vi "OutputActuators.vi"   [LabVIEW 2020]
uses:
  <vilib>/Rock Robotics/WPI/Solenoid/WPI_SolenoidValue.ctl
  cb7c92a0-f2e0-4add-9935-f208a2f5d3d6.vi
  dfd904db-942a-4b3e-8a93-2d5956c08777.vi
  05c4d3af-9fca-48dd-b3f9-451663aedd7e.vi
  outputs.vi
  TAI_Solenoid.vi
  dsdata.vi
  refnums.vi
  GRNF_GenericSolenoid.vi
  <vilib>/Rock Robotics/WPI/Solenoid/WPI_SolenoidSetEnum.vi
  <vilib>/Rock Robotics/WPI/ThirdParty/Phoenix-LabVIEW/Motor Controller/Controls/CTRE_Phoenix_MotorControl_ControlMode.ctl
  dbda877a-b90e-4fd7-958b-38a76fa4c161.vi
  GRNF_CTREMotor.vi
  TAI_Motor.vi
  cd96a094-93cf-4b37-bace-1743d092b962.vi
  3743a8f9-5793-4711-a231-b942b815bc77.vi
  c5faff8a-f8d6-4d9e-b396-3937cb23a7d4.vi
types:
  T1 = typedef "CTRE_Phoenix_MotorControl_ControlMode.ctl" = u16
  T2 = typedef "WPI_MotorControlDeviceRef.ctl" = cluster{"DeviceStatus":errorcluster, "Type":T3, "PWM":cluster{"PWM Channel":T4, "DeadBand":T5}, "CAN":cluster{"Device Number":u8, "SetOutput VI Ref":variant, "GetOutput VI Ref":variant, "Enable VI Ref":variant, "Disable VI Ref":variant, "Data":variant}, "Invert":bool, "DIO PWM":cluster{"PWM \"Enable\" Channel":T4, "DIOChannel":T6, "PWM Rate":dbl}}
  T3 = typedef "WPI_MotorControlType.ctl" = enum16{"PWM", "CAN", "DIO PWM"}
  T4 = typedef "FPGA_DIOPWMChannel.ctl" = enum8{"PWM 0", "PWM 1", "PWM 2", "PWM 3", "PWM 4", "PWM 5", "PWM 6", "PWM 7", "PWM 8", "PWM 9", "PWM MXP 0", "PWM MXP 1", "PWM MXP 2", "PWM MXP 3", "PWM MXP 4", "PWM MXP 5", "PWM MXP 6", "PWM MXP 7", "PWM MXP 8", "PWM MXP 9", "Invalid"}
  T5 = typedef "WPI_PWMDeadband.ctl" = cluster{"Name":string, "maxPositivePwm":i32, "minPositivePwm":i32, "centerPwm":i32, "maxNegativePwm":i32, "minNegativePwm":i32, "angularRange":u16}
  T6 = typedef "FPGA_DIOChannel.ctl" = enum8{"DIO 0", "DIO 1", "DIO 2", "DIO 3", "DIO 4", "DIO 5", "DIO 6", "DIO 7", "DIO 8", "DIO 9", "DIO MXP 0", "DIO MXP 1", "DIO MXP 2", "DIO MXP 3", "DIO MXP 4", "DIO MXP 5", "DIO MXP 6", "DIO MXP 7", "DIO MXP 8", "DIO MXP 9", "DIO MXP 10", "DIO MXP 11", "DIO MXP 12", "DIO MXP 13", "DIO MXP 14", "DIO MXP 15", "SPI Port CS1", "SPI Port CS2", "SPI Port CS3", "SPI Port MISO", "SPI Port MOSI", "Invalid"}
  T7 = typedef "WPI_SolenoidDevRef.ctl" = cluster{"DevStatus":errorcluster, "Pneumatics Control Module":u8, "Forward Solenoid Channel":T8, "Reverse Solenoid Channel":T8}
  T8 = typedef "WPI_SolenoidChannel.ctl" = enum8{"Solenoid 0", "Solenoid 1", "Solenoid 2", "Solenoid 3", "Solenoid 4", "Solenoid 5", "Solenoid 6", "Solenoid 7", "Solenoid 8", "Solenoid 9", "Solenoid 10", "Solenoid 11", "Solenoid 12", "Solenoid 13", "Solenoid 14", "Solenoid 15", "Invalid"}
  T9 = typedef "WPI_SolenoidValue.ctl" = enum16{"Off", "On", "Forward", "Reverse"}
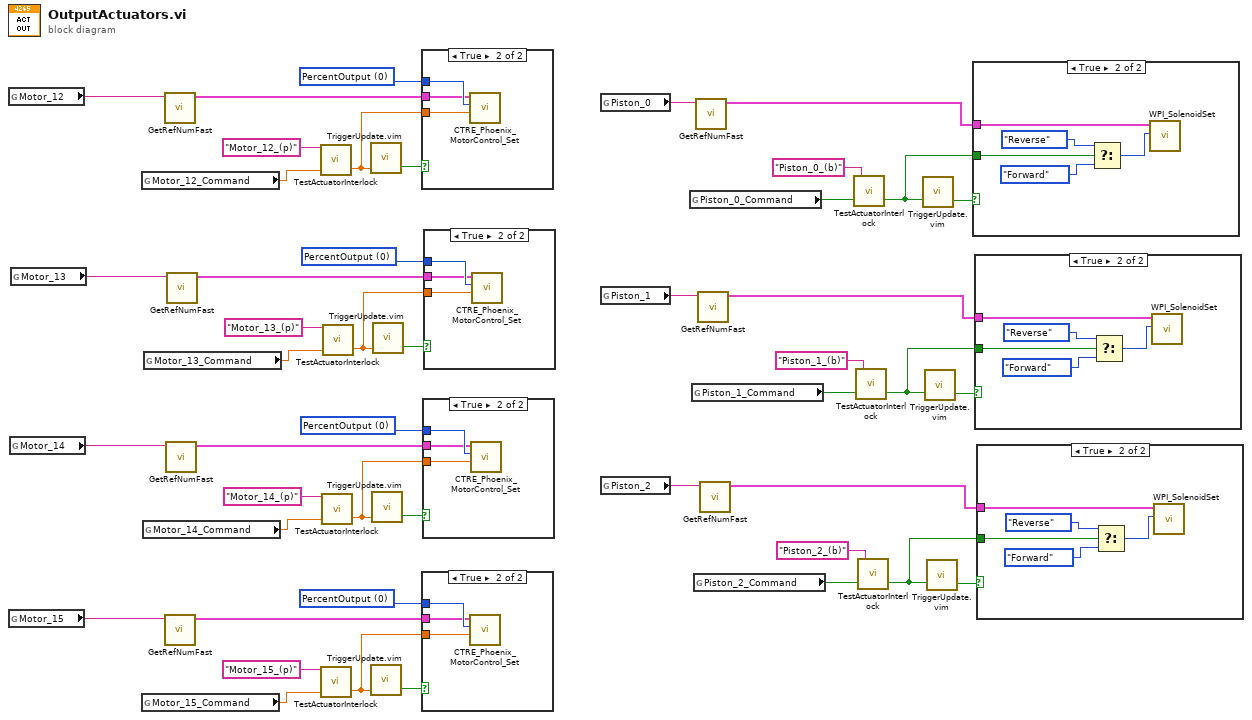
[diagram p0: block diagram]
diagram:
  w7 = T1 0 items=["PercentOutput"=0, "Position"=1, "Velocity"=2, "Current"=3, "Follower"=5, "MotionProfile"=6, "MotionMagic"=7, "MotionProfileArc"=10, "Disabled"=15] ("Control Mode")
  w14 = T1 0 items=["PercentOutput"=0, "Position"=1, "Velocity"=2, "Current"=3, "Follower"=5, "MotionProfile"=6, "MotionMagic"=7, "MotionProfileArc"=10, "Disabled"=15] ("Control Mode")
  w21 = T1 0 items=["PercentOutput"=0, "Position"=1, "Velocity"=2, "Current"=3, "Follower"=5, "MotionProfile"=6, "MotionMagic"=7, "MotionProfileArc"=10, "Disabled"=15] ("Control Mode")
  w28 = T1 0 items=["PercentOutput"=0, "Position"=1, "Velocity"=2, "Current"=3, "Follower"=5, "MotionProfile"=6, "MotionMagic"=7, "MotionProfileArc"=10, "Disabled"=15] ("Control Mode")
  n1 = global read "refnums.vi" "Motor_12"() -> (w5:string)
  n2 = global read "refnums.vi" "Motor_15"() -> (w26:string)
  n3 = global read "refnums.vi" "Motor_14"() -> (w19:string)
  n4 = global read "refnums.vi" "Motor_13"() -> (w12:string)
  n5 = global read "outputs.vi" "Motor_12_Command"() -> (w2:dbl)
  n6 = global read "outputs.vi" "Motor_15_Command"() -> (w23:dbl)
  n7 = global read "outputs.vi" "Motor_14_Command"() -> (w16:dbl)
  n8 = global read "outputs.vi" "Motor_13_Command"() -> (w9:dbl)
  n9 = call-poly "GetRefNumFast.vi"("RefNum Name"=w5) -> ("Device Reference"=w4:T2)  [unwired: 5 in, 1 out]
  n10 = call-poly "GetRefNumFast.vi"("RefNum Name"=w26) -> ("Device Reference"=w25:T2)  [unwired: 5 in, 1 out]
  n11 = call-poly "GetRefNumFast.vi"("RefNum Name"=w19) -> ("Device Reference"=w18:T2)  [unwired: 5 in, 1 out]
  n12 = call-poly "GetRefNumFast.vi"("RefNum Name"=w12) -> ("Device Reference"=w11:T2)  [unwired: 5 in, 1 out]
  n13 = call-poly "TestActuatorInterlock.vi"("Normal Output"=w2, "Actuator Name"="Motor_12_(p)") -> ("Interlock Output"=w1:dbl)  [unwired: 1 in, 1 out]
  n14 = call-poly "TestActuatorInterlock.vi"("Normal Output"=w23, "Actuator Name"="Motor_15_(p)") -> ("Interlock Output"=w22:dbl)  [unwired: 1 in, 1 out]
  n15 = call-poly "TestActuatorInterlock.vi"("Normal Output"=w16, "Actuator Name"="Motor_14_(p)") -> ("Interlock Output"=w15:dbl)  [unwired: 1 in, 1 out]
  n16 = call-poly "TestActuatorInterlock.vi"("Normal Output"=w9, "Actuator Name"="Motor_13_(p)") -> ("Interlock Output"=w8:dbl)  [unwired: 1 in, 1 out]
  n17 = call "TriggerUpdate.vim"("Trigger"=w1) -> ("Update"=w6:bool)  [unwired: 2 in]
  n18 = call "TriggerUpdate.vim"("Trigger"=w22) -> ("Update"=w27:bool)  [unwired: 2 in]
  n19 = call "TriggerUpdate.vim"("Trigger"=w15) -> ("Update"=w20:bool)  [unwired: 2 in]
  n20 = call "TriggerUpdate.vim"("Trigger"=w8) -> ("Update"=w13:bool)  [unwired: 2 in]
  n21 = case shown="True" w6 {
    tunnel: w7 -> [_ w49]
    tunnel: w4 -> [_ w48]
    tunnel: w1 -> [_ w47]
    frame False {
    }
    frame True {
      n22 = call <vilib>:"CTRE_Phoenix_MotorControl_Set.vi"("Output"=w47, "Control Mode"=w49, "PhoenixMotorControlDevRef"=w48) -> ()  [unwired: 7 in, 2 out]
    }
  }
  n23 = case shown="True" w27 {
    tunnel: w28 -> [_ w52]
    tunnel: w25 -> [_ w51]
    tunnel: w22 -> [_ w50]
    frame False {
    }
    frame True {
      n24 = call <vilib>:"CTRE_Phoenix_MotorControl_Set.vi"("Output"=w50, "Control Mode"=w52, "PhoenixMotorControlDevRef"=w51) -> ()  [unwired: 7 in, 2 out]
    }
  }
  n25 = case shown="True" w20 {
    tunnel: w21 -> [_ w55]
    tunnel: w18 -> [_ w54]
    tunnel: w15 -> [_ w53]
    frame False {
    }
    frame True {
      n26 = call <vilib>:"CTRE_Phoenix_MotorControl_Set.vi"("Output"=w53, "Control Mode"=w55, "PhoenixMotorControlDevRef"=w54) -> ()  [unwired: 7 in, 2 out]
    }
  }
  n27 = case shown="True" w13 {
    tunnel: w14 -> [_ w58]
    tunnel: w11 -> [_ w57]
    tunnel: w8 -> [_ w56]
    frame False {
    }
    frame True {
      n28 = call <vilib>:"CTRE_Phoenix_MotorControl_Set.vi"("Output"=w56, "Control Mode"=w58, "PhoenixMotorControlDevRef"=w57) -> ()  [unwired: 7 in, 2 out]
    }
  }
  n29 = global read "refnums.vi" "Piston_0"() -> (w46:string)
  n30 = global read "refnums.vi" "Piston_1"() -> (w40:string)
  n31 = global read "refnums.vi" "Piston_2"() -> (w34:string)
  n32 = global read "outputs.vi" "Piston_0_Command"() -> (w41:bool)
  n33 = global read "outputs.vi" "Piston_1_Command"() -> (w35:bool)
  n34 = global read "outputs.vi" "Piston_2_Command"() -> (w29:bool)
  n35 = call-poly "GetRefNumFast.vi"("RefNum Name"=w46) -> ("Device Reference"=w45:T7)  [unwired: 5 in, 1 out]
  n36 = call-poly "GetRefNumFast.vi"("RefNum Name"=w40) -> ("Device Reference"=w39:T7)  [unwired: 5 in, 1 out]
  n37 = call-poly "GetRefNumFast.vi"("RefNum Name"=w34) -> ("Device Reference"=w33:T7)  [unwired: 5 in, 1 out]
  n38 = call-poly "TestActuatorInterlock.vi"("Normal Output"=w41, "Actuator Name"="Piston_0_(b)") -> ("Interlock Output"=w43:bool)  [unwired: 1 in, 1 out]
  n39 = call-poly "TestActuatorInterlock.vi"("Normal Output"=w35, "Actuator Name"="Piston_1_(b)") -> ("Interlock Output"=w37:bool)  [unwired: 1 in, 1 out]
  n40 = call-poly "TestActuatorInterlock.vi"("Normal Output"=w29, "Actuator Name"="Piston_2_(b)") -> ("Interlock Output"=w31:bool)  [unwired: 1 in, 1 out]
  n41 = call "TriggerUpdate.vim"("Trigger"=w43) -> ("Update"=w44:bool)  [unwired: 2 in]
  n42 = call "TriggerUpdate.vim"("Trigger"=w37) -> ("Update"=w38:bool)  [unwired: 2 in]
  n43 = call "TriggerUpdate.vim"("Trigger"=w31) -> ("Update"=w32:bool)  [unwired: 2 in]
  n44 = case shown="True" w44 {
    tunnel: w45 -> [_ w63]
    tunnel: w43 -> [_ w62]
    frame False {
    }
    frame True {
      n45 = Select(t=WPI_SolenoidValue."Reverse" ("Value"), s=w62, f=WPI_SolenoidValue."Forward" ("Value")) -> (s? t:f=w61:T9)
      n46 = call-poly <vilib>:"WPI_SolenoidSet.vi"("Value"=w61, "SolenoidDevRef"=w63) -> ()  [unwired: 8 in, 2 out]
    }
  }
  n47 = case shown="True" w38 {
    tunnel: w39 -> [_ w68]
    tunnel: w37 -> [_ w67]
    frame False {
    }
    frame True {
      n48 = Select(t=WPI_SolenoidValue."Reverse" ("Value"), s=w67, f=WPI_SolenoidValue."Forward" ("Value")) -> (s? t:f=w66:T9)
      n49 = call-poly <vilib>:"WPI_SolenoidSet.vi"("Value"=w66, "SolenoidDevRef"=w68) -> ()  [unwired: 8 in, 2 out]
    }
  }
  n50 = case shown="True" w32 {
    tunnel: w33 -> [_ w73]
    tunnel: w31 -> [_ w72]
    frame False {
    }
    frame True {
      n51 = Select(t=WPI_SolenoidValue."Reverse" ("Value"), s=w72, f=WPI_SolenoidValue."Forward" ("Value")) -> (s? t:f=w71:T9)
      n52 = call-poly <vilib>:"WPI_SolenoidSet.vi"("Value"=w71, "SolenoidDevRef"=w73) -> ()  [unwired: 8 in, 2 out]
    }
  }
